vi "publish_status.vi"() -> ()   [LabVIEW 2018]
uses:
  RxTx/RxTx.lvclass
  <vilib>/addons/zeromq/socket_type.ctl
  <vilib>/addons/zeromq/zmq_socket.lvclass
  <vilib>/addons/zeromq/zmq_context.lvclass
  <vilib>/addons/zeromq/zeromq.lvlib
panel:
  in  "Stop Button 5":bool
  in  "Stop Button 4":bool
  in  "RxTx.lvclass 3":refnum<class "RxTx.lvclass">
  in  "Stop Button 3":bool
  in  "Stop Button 2":bool
  in  "Stop Button":bool
  out "error out 3":errorcluster
  in  "RxTx.lvclass 2":refnum<class "RxTx.lvclass">
  # "Channel 1 - ZEROMQ Communication"
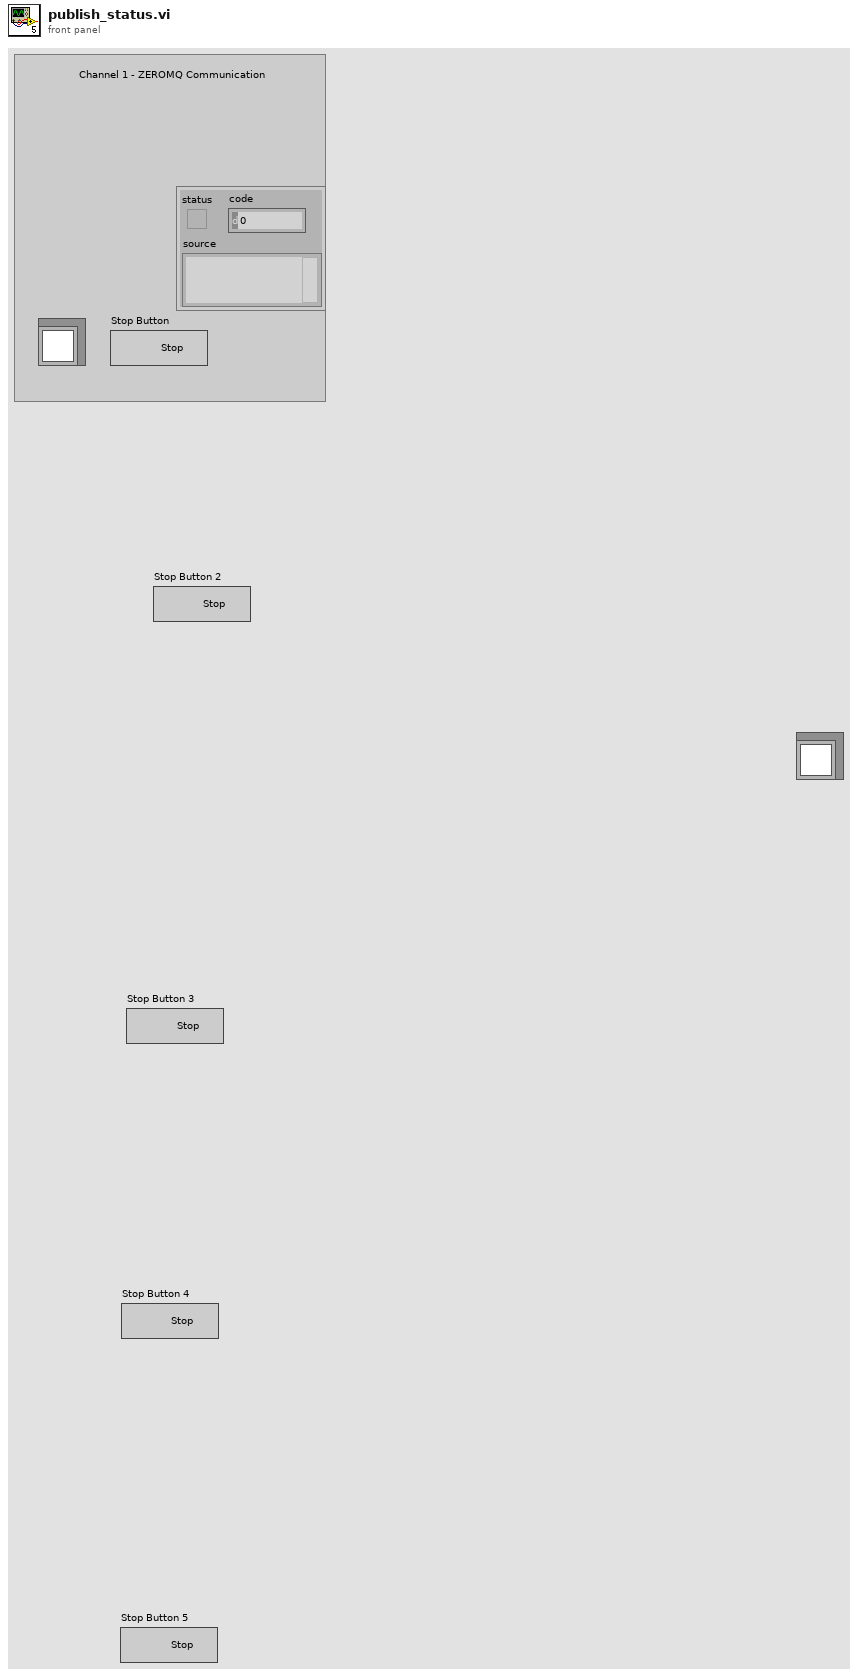
[diagram p1: front panel]
types:
  T1 = typedef "zeromq.lvlib/socket_type.ctl" = enum8{"ZMQ_PAIR", "ZMQ_PUB", "ZMQ_SUB", "ZMQ_REQ", "ZMQ_REP", "ZMQ_DEALER", "ZMQ_ROUTER", "ZMQ_PULL", "ZMQ_PUSH", "ZMQ_XPUB", "ZMQ_XSUB", "ZMQ_STREAM", "ZMQ_SERVER", "ZMQ_CLIENT", "ZMQ_RADIO", "ZMQ_DISH", "ZMQ_GATHER", "ZMQ_SCATTER", "ZMQ_DGRAM"}
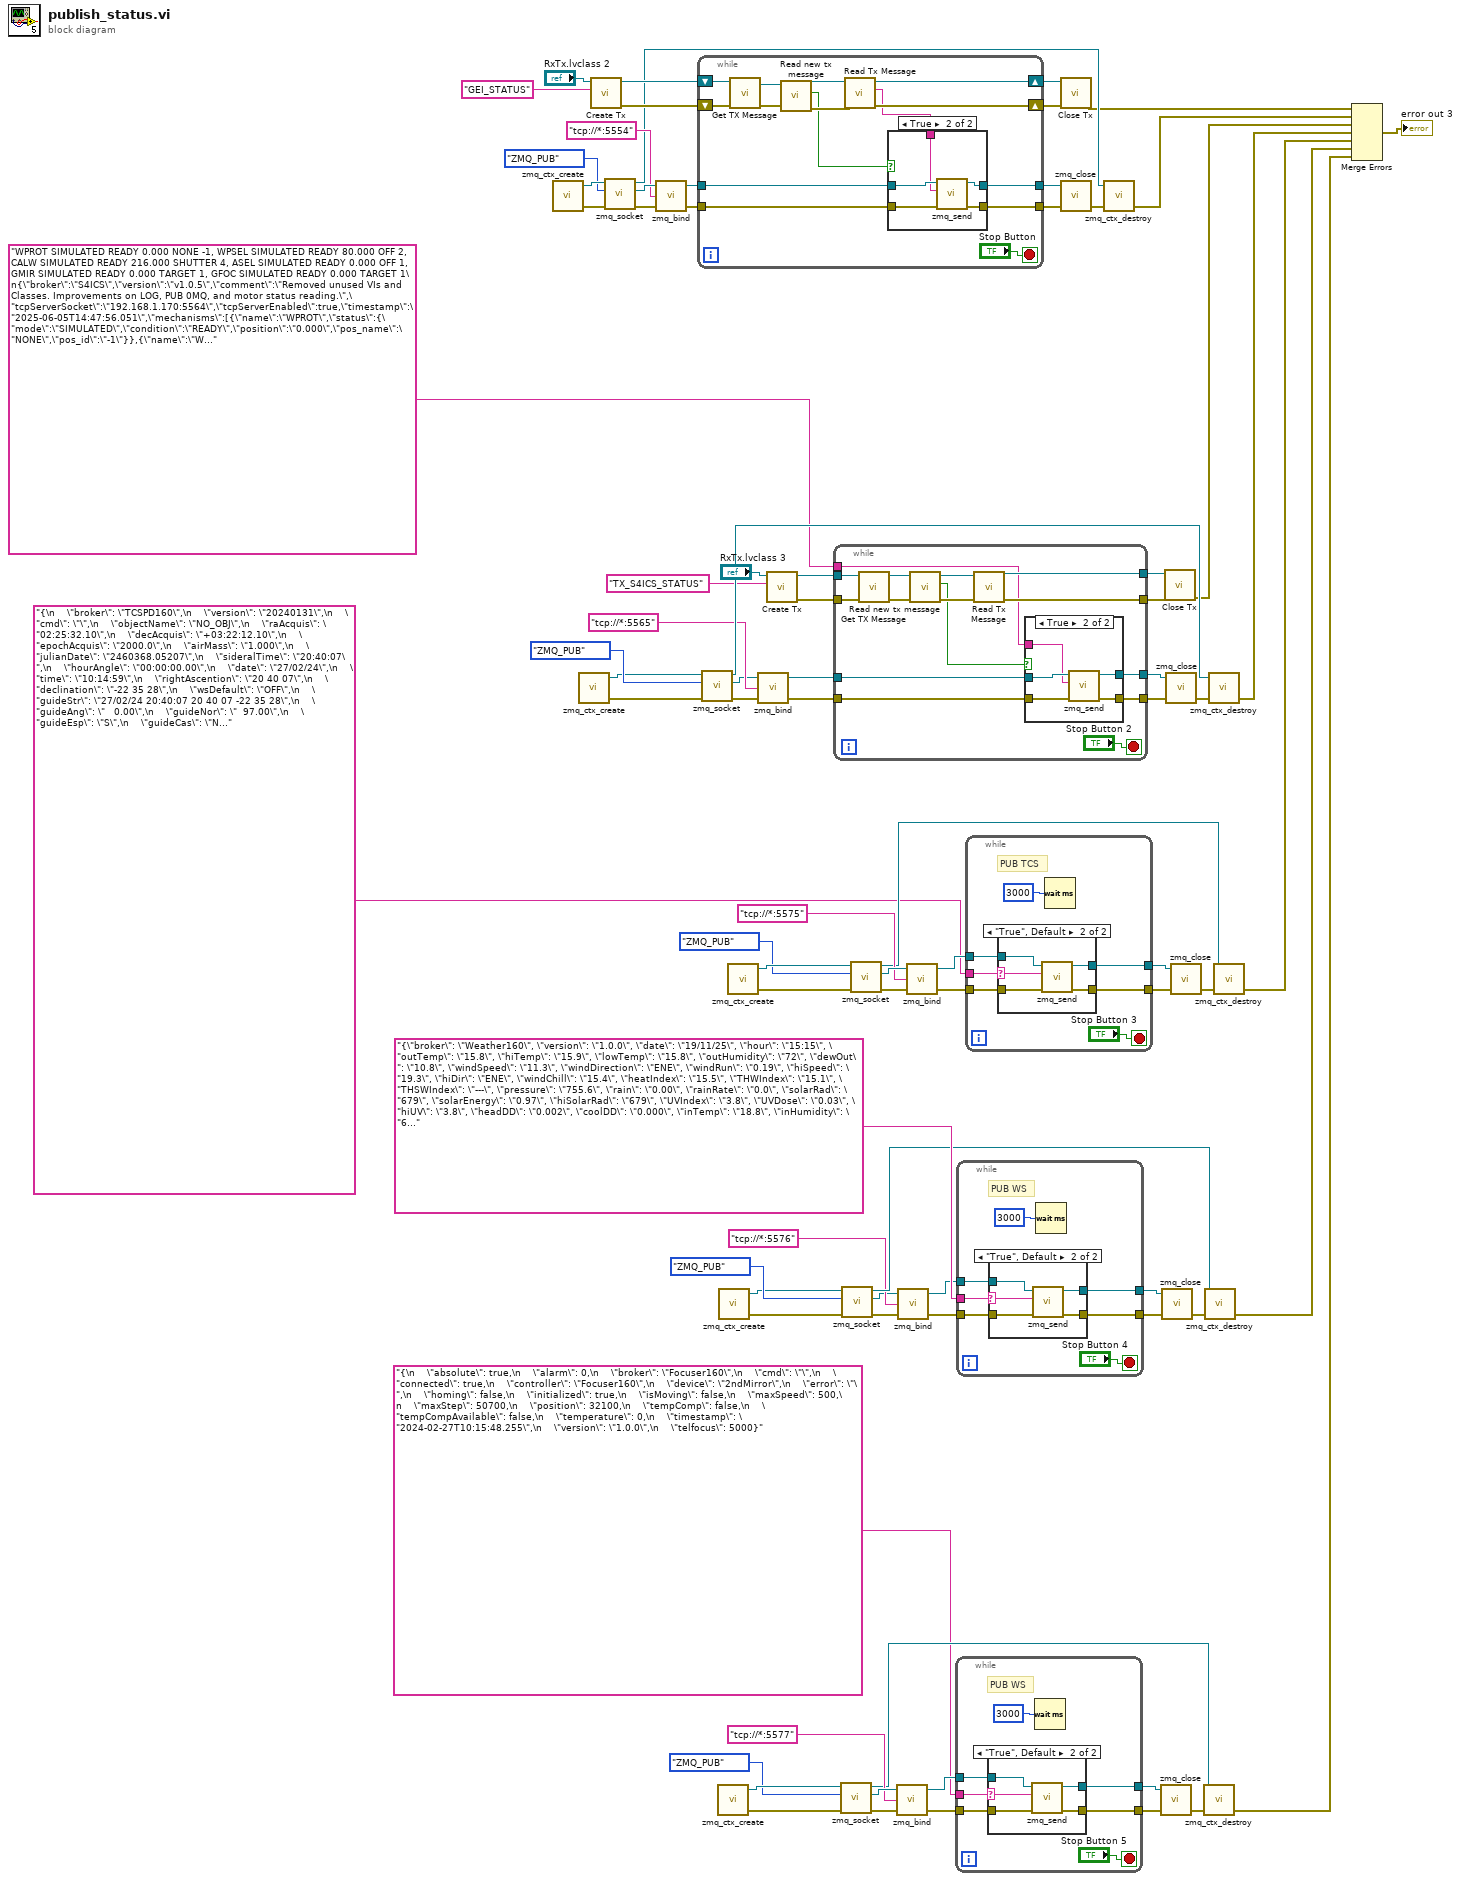
[diagram p0: block diagram]
diagram:
  n1 = call <vilib>:"zmq_ctx_create.vi"() -> ("error out"=w76:errorcluster, "context out"=w79:refnum<class "zmq_context.lvclass">)  [unwired: 4 in]
  n2 = call <vilib>:"zmq_ctx_create.vi"() -> ("error out"=w58:errorcluster, "context out"=w55:refnum<class "zmq_context.lvclass">)  [unwired: 4 in]
  n3 = call "Create Tx.vi"("Writer Name"="GEI_STATUS" ("string"), "RxTx in"="RxTx.lvclass 2") -> ("error out"=w81:errorcluster, "RxTx out"=w82:refnum<class "RxTx.lvclass">)  [unwired: 8 in]
  n4 = call <vilib>:"zmq_socket.vi"("error in"=w76, "socket type"=socket_type."ZMQ_PUB", "context in"=w79) -> ("error out"=w78:errorcluster, "socket out"=w77:refnum<class "zmq_socket.lvclass">, "context out"=w70:refnum<class "zmq_context.lvclass">)  [unwired: 2 in]
  n5 = call <vilib>:"zmq_bind.vi"("error in"=w78, "endpoint"="tcp://*:5554", "socket in"=w77) -> ("error out"=w71:errorcluster, "socket out"=w72:refnum<class "zmq_socket.lvclass">)  [unwired: 1 in]
  n6 = while {
    shift-right: [w99] -> w84
    shift-left: w82 -> [w98]
    shift-right: [w96] -> w80
    shift-left: w81 -> [w97]
    tunnel: w72 -> [w95]
    tunnel: w71 -> [w94]
    tunnel: [w93] -> w69
    tunnel: [w92] -> w68
    stop <- "Stop Button" stop-if-true
    n7 = call "Get TX Message.vi"("error in (no error)"=w97, "RxTx in"=w98) -> ("error out"=w90:errorcluster, "RxTx out"=w87:refnum<class "RxTx.lvclass">)  [unwired: 8 in]
    n8 = call-dynamic "Read new tx message.vi"("error in (no error)"=w90, "RxTx in"=w87) -> ("error out"=w89:errorcluster, "new tx message"=w86:bool, "RxTx out"=w88:refnum<class "RxTx.lvclass">)  [unwired: 7 in]
    n9 = call "Read Tx Message.vi"("error in (no error)"=w89, "RxTx in"=w88) -> ("error out"=w96:errorcluster, "Tx Message"=w85:string, "RxTx out"=w99:refnum<class "RxTx.lvclass">)  [unwired: 7 in]
    n10 = case shown="True" w86 {
      tunnel: w95 -> [w101 w106]
      tunnel: w94 -> [w100 w105]
      tunnel: [w101 w104] -> w93
      tunnel: [w100 w103] -> w92
      tunnel: w85 -> [_ w102]
      frame False {
      }
      frame True, Default {
        n11 = call <vilib>:"zmq_send.vi"("error in"=w105, "data"=w102, "socket in"=w106) -> ("error out"=w103:errorcluster, "socket out"=w104:refnum<class "zmq_socket.lvclass">)  [unwired: 4 in]
      }
    }
  }
  n12 = call <vilib>:"zmq_socket.vi"("error in"=w58, "socket type"=socket_type."ZMQ_PUB", "context in"=w55) -> ("error out"=w56:errorcluster, "socket out"=w57:refnum<class "zmq_socket.lvclass">, "context out"=w64:refnum<class "zmq_context.lvclass">)  [unwired: 2 in]
  n13 = call <vilib>:"zmq_ctx_create.vi"() -> ("error out"=w11:errorcluster, "context out"=w14:refnum<class "zmq_context.lvclass">)  [unwired: 4 in]
  n14 = call <vilib>:"zmq_ctx_create.vi"() -> ("error out"=w19:errorcluster, "context out"=w16:refnum<class "zmq_context.lvclass">)  [unwired: 4 in]
  n15 = call <vilib>:"zmq_ctx_create.vi"() -> ("error out"=w51:errorcluster, "context out"=w54:refnum<class "zmq_context.lvclass">)  [unwired: 4 in]
  n16 = call <vilib>:"zmq_bind.vi"("error in"=w56, "endpoint"="tcp://*:5565", "socket in"=w57) -> ("error out"=w63:errorcluster, "socket out"=w62:refnum<class "zmq_socket.lvclass">)  [unwired: 1 in]
  n17 = call "Create Tx.vi"("Writer Name"="TX_S4ICS_STATUS" ("string"), "RxTx in"="RxTx.lvclass 3") -> ("error out"=w35:errorcluster, "RxTx out"=w36:refnum<class "RxTx.lvclass">)  [unwired: 8 in]
  n18 = while {
    tunnel: w62 -> [w121]
    tunnel: w63 -> [w120]
    tunnel: [w119] -> w65
    tunnel: [w118] -> w66
    tunnel: "WPROT SIMULATED READY 0.000 NONE -1, WPSEL SIMULATED READY 80.000 OFF 2, CALW SIMULATED READY 216.000 SHUTTER 4, ASEL SIMULATED READY 0.000 OFF 1, GMIR SIMULATED READY 0.000 TARGET 1, GFOC SIMULATED READY 0.000 TARGET 1\n{\"broker\":\"S4ICS\",\"version\":\"v1.0.5\",\"comment\":\"Removed unused VIs and Classes. Improvements on LOG, PUB 0MQ, and motor status reading.\",\"tcpServerSocket\":\"192.168.1.170:5564\",\"tcpServerEnabled\":true,\"timestamp\":\"2025-06-05T14:47:56.051\",\"mechanisms\":[{\"name\":\"WPROT\",\"status\":{\"mode\":\"SIMULATED\",\"condition\":\"READY\",\"position\":\"0.000\",\"pos_name\":\"NONE\",\"pos_id\":\"-1\"}},{\"name\":\"WPSEL\",\"status\":{\"mode\":\"SIMULATED\",\"condition\":\"READY\",\"position\":\"80.000\",\"pos_name\":\"OFF\",\"pos_id\":\"2\"}},{\"name\":\"CALW\",\"status\":{\"mode\":\"SIMULATED\",\"condition\":\"READY\",\"position\":\"216.000\",\"pos_name\":\"CLOSED\",\"pos_id\":\"4\"}},{\"name\":\"ASEL\",\"status\":{\"mode\":\"SIMULATED\",\"condition\":\"READY\",\"position\":\"0.000\",\"pos_name\":\"OFF\",\"pos_id\":\"1\"}},{\"name\":\"GMIR\",\"status\":{\"mode\":\"SIMULATED\",\"condition\":\"READY\",\"position\":\"0.000\",\"pos_name\":\"TARGET\",\"pos_id\":\"1\"}},{\"name\":\"GFOC\",\"status\":{\"mode\":\"SIMULATED\",\"condition\":\"READY\",\"position\":\"8.0\",\"pos_name\":\"TARGET\",\"pos_id\":\"-1\"}}]}" ("endpoint") -> [w107]
    tunnel: [w111] -> w38
    tunnel: [w110] -> w37
    tunnel: w36 -> [w109]
    tunnel: w35 -> [w108]
    stop <- "Stop Button 2" stop-if-true
    n19 = call "Get TX Message.vi"("error in (no error)"=w108, "RxTx in"=w109) -> ("error out"=w116:errorcluster, "RxTx out"=w113:refnum<class "RxTx.lvclass">)  [unwired: 8 in]
    n20 = call-dynamic "Read new tx message.vi"("error in (no error)"=w116, "RxTx in"=w113) -> ("error out"=w115:errorcluster, "new tx message"=w112:bool, "RxTx out"=w114:refnum<class "RxTx.lvclass">)  [unwired: 7 in]
    n21 = call "Read Tx Message.vi"("error in (no error)"=w115, "RxTx in"=w114) -> ("error out"=w111:errorcluster, "RxTx out"=w110:refnum<class "RxTx.lvclass">)  [unwired: 7 in, 1 out]
    n22 = case shown="True" w112 {
      tunnel: w121 -> [w123 w128]
      tunnel: w120 -> [w122 w127]
      tunnel: [w123 w126] -> w119
      tunnel: [w122 w125] -> w118
      tunnel: w107 -> [_ w124]
      frame False {
      }
      frame True, Default {
        n23 = call <vilib>:"zmq_send.vi"("error in"=w127, "data"=w124, "socket in"=w128) -> ("error out"=w125:errorcluster, "socket out"=w126:refnum<class "zmq_socket.lvclass">)  [unwired: 4 in]
      }
    }
  }
  n24 = call <vilib>:"zmq_socket.vi"("error in"=w11, "socket type"=socket_type."ZMQ_PUB", "context in"=w14) -> ("error out"=w13:errorcluster, "socket out"=w12:refnum<class "zmq_socket.lvclass">, "context out"=w5:refnum<class "zmq_context.lvclass">)  [unwired: 2 in]
  n25 = call <vilib>:"zmq_socket.vi"("error in"=w19, "socket type"=socket_type."ZMQ_PUB", "context in"=w16) -> ("error out"=w17:errorcluster, "socket out"=w18:refnum<class "zmq_socket.lvclass">, "context out"=w25:refnum<class "zmq_context.lvclass">)  [unwired: 2 in]
  n26 = call <vilib>:"zmq_socket.vi"("error in"=w51, "socket type"=socket_type."ZMQ_PUB", "context in"=w54) -> ("error out"=w53:errorcluster, "socket out"=w52:refnum<class "zmq_socket.lvclass">, "context out"=w45:refnum<class "zmq_context.lvclass">)  [unwired: 2 in]
  n27 = call <vilib>:"zmq_bind.vi"("error in"=w13, "endpoint"="tcp://*:5577", "socket in"=w12) -> ("error out"=w6:errorcluster, "socket out"=w7:refnum<class "zmq_socket.lvclass">)  [unwired: 1 in]
  n28 = call <vilib>:"zmq_bind.vi"("error in"=w17, "endpoint"="tcp://*:5576", "socket in"=w18) -> ("error out"=w24:errorcluster, "socket out"=w23:refnum<class "zmq_socket.lvclass">)  [unwired: 1 in]
  n29 = call <vilib>:"zmq_bind.vi"("error in"=w53, "endpoint"="tcp://*:5575", "socket in"=w52) -> ("error out"=w46:errorcluster, "socket out"=w47:refnum<class "zmq_socket.lvclass">)  [unwired: 1 in]
  n30 = while {
    tunnel: w7 -> [w135]
    tunnel: w6 -> [w134]
    tunnel: [w133] -> w4
    tunnel: [w132] -> w3
    tunnel: "{\n    \"absolute\": true,\n    \"alarm\": 0,\n    \"broker\": \"Focuser160\",\n    \"cmd\": \"\",\n    \"connected\": true,\n    \"controller\": \"Focuser160\",\n    \"device\": \"2ndMirror\",\n    \"error\": \"\",\n    \"homing\": false,\n    \"initialized\": true,\n    \"isMoving\": false,\n    \"maxSpeed\": 500,\n    \"maxStep\": 50700,\n    \"position\": 32100,\n    \"tempComp\": false,\n    \"tempCompAvailable\": false,\n    \"temperature\": 0,\n    \"timestamp\": \"2024-02-27T10:15:48.255\",\n    \"version\": \"1.0.0\",\n    \"telfocus\": 5000}" ("endpoint") -> [w130]
    stop <- "Stop Button 5" stop-if-true
    # "PUB WS"
    n31 = case shown="\"True\", Default" w130 {
      selector: w130 -> [_ w138]
      tunnel: w135 -> [w137 w142]
      tunnel: w134 -> [w136 w141]
      tunnel: [w137 w140] -> w133
      tunnel: [w136 w139] -> w132
      frame "", "STOP_APPLICATION" {
      }
      frame "True", Default {
        n32 = call <vilib>:"zmq_send.vi"("error in"=w141, "data"=w138, "socket in"=w142) -> ("error out"=w139:errorcluster, "socket out"=w140:refnum<class "zmq_socket.lvclass">)  [unwired: 4 in]
      }
    }
    n33 = Wait (ms)(milliseconds to wait=u32 3000) -> ()  [unwired: 1 out]
  }
  n34 = while {
    tunnel: w23 -> [w149]
    tunnel: w24 -> [w148]
    tunnel: [w147] -> w26
    tunnel: [w146] -> w27
    tunnel: "{\"broker\": \"Weather160\", \"version\": \"1.0.0\", \"date\": \"19/11/25\", \"hour\": \"15:15\", \"outTemp\": \"15.8\", \"hiTemp\": \"15.9\", \"lowTemp\": \"15.8\", \"outHumidity\": \"72\", \"dewOut\": \"10.8\", \"windSpeed\": \"11.3\", \"windDirection\": \"ENE\", \"windRun\": \"0.19\", \"hiSpeed\": \"19.3\", \"hiDir\": \"ENE\", \"windChill\": \"15.4\", \"heatIndex\": \"15.5\", \"THWIndex\": \"15.1\", \"THSWIndex\": \"---\", \"pressure\": \"755.6\", \"rain\": \"0.00\", \"rainRate\": \"0.0\", \"solarRad\": \"679\", \"solarEnergy\": \"0.97\", \"hiSolarRad\": \"679\", \"UVIndex\": \"3.8\", \"UVDose\": \"0.03\", \"hiUV\": \"3.8\", \"headDD\": \"0.002\", \"coolDD\": \"0.000\", \"inTemp\": \"18.8\", \"inHumidity\": \"63\", \"dewIn\": \"11.6\", \"inHeat\": \"18.4\", \"inEMC\": \"11.63\", \"inAirDensity\": \"1.1865\", \"2ndTemp\": \"20.0\", \"2ndHumidity\": \"50\", \"ET\": \"0.00\", \"leaf\": \"0\", \"windSamp\": \"22\", \"windTx\": \"1\", \"ISSRecept\": \"95.7\", \"arcInt\": \"1\"}" ("endpoint") -> [w144]
    stop <- "Stop Button 4" stop-if-true
    # "PUB WS"
    n35 = case shown="\"True\", Default" w144 {
      selector: w144 -> [_ w152]
      tunnel: w149 -> [w151 w156]
      tunnel: w148 -> [w150 w155]
      tunnel: [w151 w154] -> w147
      tunnel: [w150 w153] -> w146
      frame "", "STOP_APPLICATION" {
      }
      frame "True", Default {
        n36 = call <vilib>:"zmq_send.vi"("error in"=w155, "data"=w152, "socket in"=w156) -> ("error out"=w153:errorcluster, "socket out"=w154:refnum<class "zmq_socket.lvclass">)  [unwired: 4 in]
      }
    }
    n37 = Wait (ms)(milliseconds to wait=u32 3000) -> ()  [unwired: 1 out]
  }
  n38 = while {
    tunnel: w47 -> [w163]
    tunnel: w46 -> [w162]
    tunnel: [w161] -> w44
    tunnel: [w160] -> w43
    tunnel: "{\n    \"broker\": \"TCSPD160\",\n    \"version\": \"20240131\",\n    \"cmd\": \"\",\n    \"objectName\": \"NO_OBJ\",\n    \"raAcquis\": \"02:25:32.10\",\n    \"decAcquis\": \"+03:22:12.10\",\n    \"epochAcquis\": \"2000.0\",\n    \"airMass\": \"1.000\",\n    \"julianDate\": \"2460368.05207\",\n    \"sideralTime\": \"20:40:07\",\n    \"hourAngle\": \"00:00:00.00\",\n    \"date\": \"27/02/24\",\n    \"time\": \"10:14:59\",\n    \"rightAscention\": \"20 40 07\",\n    \"declination\": \"-22 35 28\",\n    \"wsDefault\": \"OFF\",\n    \"guideStr\": \"27/02/24 20:40:07 20 40 07 -22 35 28\",\n    \"guideAng\": \"   0.00\",\n    \"guideNor\": \"  97.00\",\n    \"guideEsp\": \"S\",\n    \"guideCas\": \"N\",\n    \"guidePlaca\": \"0.091\",\n    \"statShutter\": \"\",\n    \"posCup\": \"\",\n    \"raOnTarget\": true,\n    \"decOnTarget\": true,\n    \"dome\": false,\n    \"domeOnTarget\": true,\n    \"guider\": false,\n    \"mount\": false,\n    \"grossMovement\": false,\n    \"fineMovement\": false,\n    \"objCentrado\": false,\n    \"varTracking\": false,\n    \"shutter\": false}" ("endpoint") -> [w158]
    stop <- "Stop Button 3" stop-if-true
    # "PUB TCS"
    n39 = case shown="\"True\", Default" w158 {
      selector: w158 -> [_ w166]
      tunnel: w163 -> [w165 w170]
      tunnel: w162 -> [w164 w169]
      tunnel: [w165 w168] -> w161
      tunnel: [w164 w167] -> w160
      frame "", "STOP_APPLICATION" {
      }
      frame "True", Default {
        n40 = call <vilib>:"zmq_send.vi"("error in"=w169, "data"=w166, "socket in"=w170) -> ("error out"=w167:errorcluster, "socket out"=w168:refnum<class "zmq_socket.lvclass">)  [unwired: 4 in]
      }
    }
    n41 = Wait (ms)(milliseconds to wait=u32 3000) -> ()  [unwired: 1 out]
  }
  n42 = call "Close Tx.vi"("error in (no error)"=w80, "RxTx in"=w84) -> ("error out"=w33:errorcluster)  [unwired: 8 in, 1 out]
  n43 = call <vilib>:"zmq_close.vi"("error in"=w68, "socket"=w69) -> ("error out"=w73:errorcluster)  [unwired: 3 in]
  n44 = call <vilib>:"zmq_ctx_destroy.vi"("error in"=w73, "context in"=w70) -> ("error out"=w32:errorcluster)  [unwired: 3 in]
  n45 = call <vilib>:"zmq_close.vi"("error in"=w3, "socket"=w4) -> ("error out"=w8:errorcluster)  [unwired: 3 in]
  n46 = call <vilib>:"zmq_close.vi"("error in"=w27, "socket"=w26) -> ("error out"=w22:errorcluster)  [unwired: 3 in]
  n47 = call "Close Tx.vi"("error in (no error)"=w38, "RxTx in"=w37) -> ("error out"=w29:errorcluster)  [unwired: 8 in, 1 out]
  n48 = call <vilib>:"zmq_close.vi"("error in"=w66, "socket"=w65) -> ("error out"=w61:errorcluster)  [unwired: 3 in]
  n49 = call <vilib>:"zmq_close.vi"("error in"=w43, "socket"=w44) -> ("error out"=w48:errorcluster)  [unwired: 3 in]
  n50 = call <vilib>:"zmq_ctx_destroy.vi"("error in"=w8, "context in"=w5) -> ("error out"=w1:errorcluster)  [unwired: 3 in]
  n51 = call <vilib>:"zmq_ctx_destroy.vi"("error in"=w22, "context in"=w25) -> ("error out"=w15:errorcluster)  [unwired: 3 in]
  n52 = call <vilib>:"zmq_ctx_destroy.vi"("error in"=w61, "context in"=w64) -> ("error out"=w31:errorcluster)  [unwired: 3 in]
  n53 = call <vilib>:"zmq_ctx_destroy.vi"("error in"=w48, "context in"=w45) -> ("error out"=w30:errorcluster)  [unwired: 3 in]
  n54 = Merge Errors(w33, w32, w29, w31, w30, w15, w1) -> (→"error out 3":errorcluster)
